vi "Add Graphic to Collection.vi"(8 "Graphic":refnum<class "Graphic.lvclass">, 11 "Collection of Graphics In":refnum<class "Collection.lvclass">) -> (3 "Collection of Graphics Out":refnum<class "Collection.lvclass">)   [LabVIEW 2023, in "Collection.lvclass"]
doc: "Add graphic to collection."
uses:
  Collection.lvclass
  c:/dev/_r/4/eng/lv-core/lvpostprocessingd/lv_mc_x86_64/dist_i386/examples/Object-Oriented Programming/Graphics/Graphic/Graphic.lvclass
  Graphic/Graphic.lvclass
  Collection.lvclass/Collection.ctl
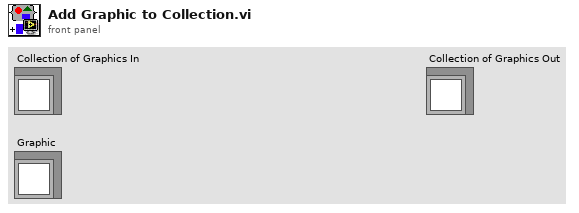
[diagram p1: front panel]
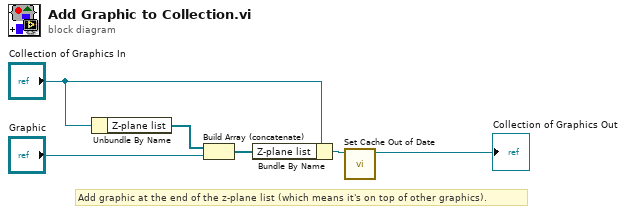
[diagram p0: block diagram]
diagram:
  # "Add graphic at the end of the z-plane list (which means it's on top of other graphics)."
  n1 = Unbundle By Name("Collection of Graphics In") -> ("Z-plane list"=w6:refnum<class "Graphic.lvclass">[])
  n2 = Build Array (concatenate)(w6, "Graphic") -> (w3:refnum<class "Graphic.lvclass">[])
  n3 = Bundle By Name(cluster="Collection of Graphics In", "Z-plane list"=w3) -> (w2:refnum<class "Collection.lvclass">)
  n4 = call "Set Cache Out of Date.vi"("Graphic.lvclass"=w2) -> ("Graphic.lvclass out"=→"Collection of Graphics Out":refnum<class "Collection.lvclass">)  [unwired: 10 in]
